vi "setSumWaveform.vi"(7 "Waveform":enum16{"Sine", "Rectangular", "Triangular"}(ring), 8 "error in (no error)":errorcluster, 9 "Frequency [Hz]":dbl, 10 "Amplitude [%]":dbl, 11 "VISA resource name":refnum<visa-resource-name>) -> (0 "error out":errorcluster, 3 "VISA resource name out":refnum<visa-resource-name>)   [LabVIEW 2023, in "Keysight-33500B.lvlib"]
doc: "<b>Author:</b> Wolfgang\n<b>Description:</b>The SUM subsystem adds a modulation source signal to a channel's primary signal. This allows you to generate a two-tone signal on one channel, or to add noise to a primary signal. The SUM function uses the same secondary sources as used by the modulation subsystems."
uses:
  Keysight-33500B.lvlib
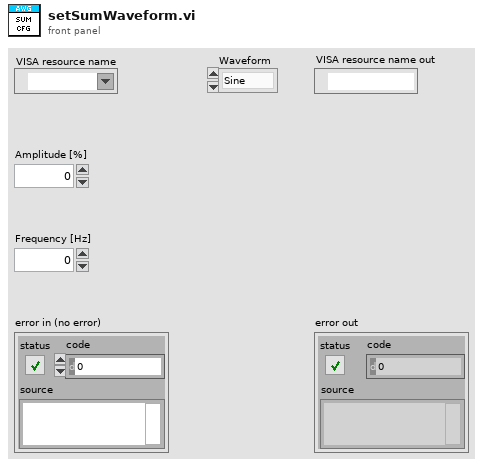
[diagram p1: front panel]
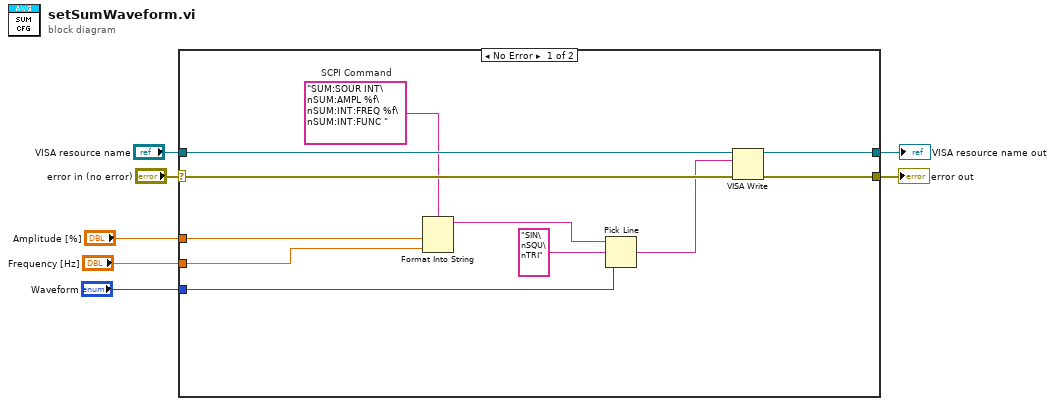
[diagram p0: block diagram]
diagram:
  n1 = case shown="No Error" "error in (no error)" {
    selector: "error in (no error)" -> [w15 w20]
    tunnel: [w17 w19] -> w7
    tunnel: [w18 w20] -> w5
    tunnel: "VISA resource name" -> [w16 w19]
    tunnel: "Amplitude [%]" -> [w14 _]
    tunnel: "Frequency [Hz]" -> [w13 _]
    tunnel: "Waveform" -> [w8 _]
    frame No Error {
      w12 = "SUM:SOUR INT\nSUM:AMPL %f\nSUM:INT:FREQ %f\nSUM:INT:FUNC "  # SCPI Command
      n2 = Format Into String(format string=w12, w14, w13) -> (resulting string=w10:string)  [unwired: 2 in, 1 out]
      n3 = Pick Line(string ("")=w10, multi-line string="SIN\nSQU\nTRI", line index=w8) -> (output string=w11:string)
      n4 = VISA Write(VISA resource name=w16, write buffer=w11, error in (no error)=w15) -> (VISA resource name out=w17:refnum<visa-resource-name>, error out=w18:errorcluster)  [unwired: 1 out]
    }
    frame Error {
    }
  }
  "VISA resource name out" <- w7
  "error out" <- w5
